vi "_WSASocket.vi"(8 "Error In":errorcluster) -> (0 "Error Out":errorcluster, 3 "Socket":u32 format="%08x")   [LabVIEW 2018]
uses:
  ws2_32.dll
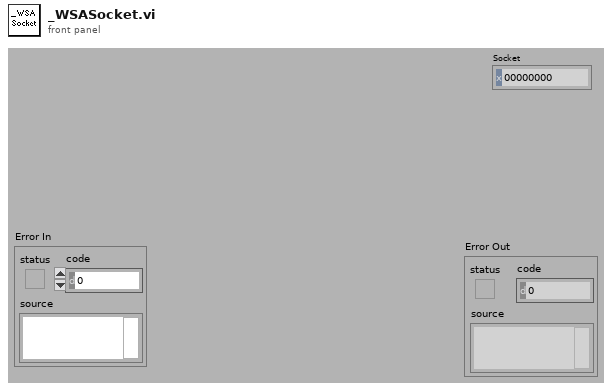
[diagram p1: front panel]
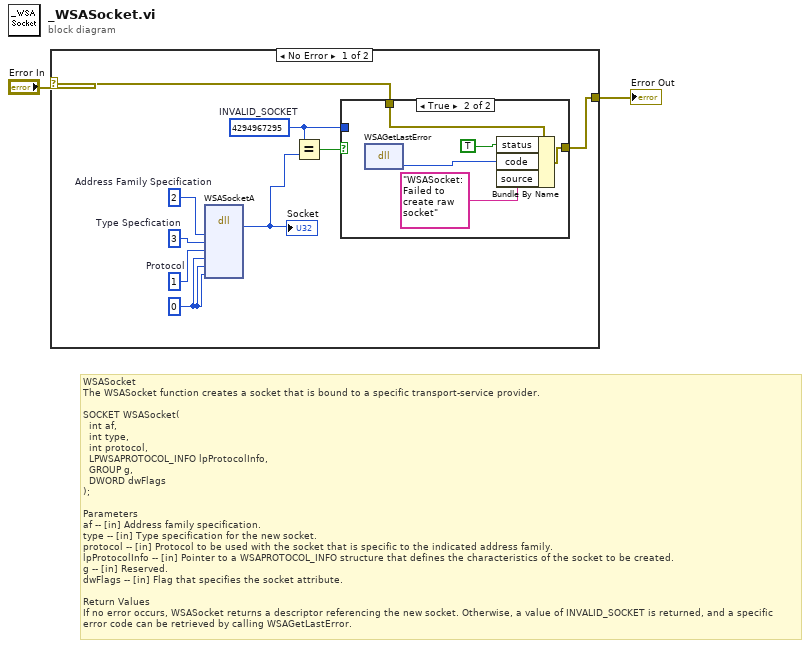
[diagram p0: block diagram]
diagram:
  # "WSASocket\nThe WSASocket function creates a socket that is bound to a specific transport-service provider.\n\nSOCKET WSASocket(\n  int af,\n  int type,\n  int protocol,\n  LPWSAPROTOCOL_INFO lpProtocolInfo,\n  GROUP g,\n  DWORD dwFlags\n);\n\nParameters\naf -- [in] Address family specification. \ntype -- [in] Type specification for the new socket. \nprotocol -- [in] Protocol to be used with the socket that is specific to the indicated address family. \nlpProtocolInfo -- [in] Pointer to a WSAPROTOCOL_INFO structure that defines the characteristics of the socket to be created. \ng -- [in] Reserved. \ndwFlags -- [in] Flag that specifies the socket attribute. \n\nReturn Values\nIf no error occurs, WSASocket returns a descriptor referencing the new socket. Otherwise, a value of INVALID_SOCKET is returned, and a specific error code can be retrieved by calling WSAGetLastError."
  n1 = case shown="No Error" "Error In" {
    selector: "Error In" -> [w5 w18]
    tunnel: [w4 w18] -> w1
    frame No Error {
      w3 = u32 4294967295  # INVALID_SOCKET
      w11 = u32 1  # Protocol
      w9 = u32 3  # Type Specfication
      w10 = u32 2  # Address Family Specification
      w8 = u32 0 ("dwFlags")
      n2 = dll-call lib="ws2_32.dll" fn="WSASocketA" label="WSASocket"("Address Family Specification"=w10, "Type Specfication"=w9, "Protocol"=w11, "lpProtocolInfo"=w8, "Group"=w8, "dwFlags"=w8) -> ("socket"=w7:u32)  [unwired: 9 in, 2 out]
      "Socket" <- w7
      n3 = Equal?(x=w3, y=w7) -> (x = y?=w6:bool)
      n4 = case shown="True" w6 {
        tunnel: w5 -> [w12 w17]
        tunnel: [w12 w16] -> w4
        tunnel: w3 -> [_ _]
        frame False {
        }
        frame True {
          n5 = dll-call lib="ws2_32.dll" fn="WSAGetLastError"() -> (w13:i32)  [unwired: 3 in, 2 out]
          n6 = Bundle By Name(cluster=w17, "status"=TRUE, "code"=w13, "source"="WSASocket: Failed to create raw socket") -> (w16:errorcluster)
        }
      }
    }
    frame Error {
    }
  }
  "Error Out" <- w1
